vi "Word_Set_Page_Numbering.vi"(7 "Include total pages":bool, 8 "error in (no error)":errorcluster, 10 "alignment (right)":u16, 11 "report in":refnum<class "NI_report.lvclass">) -> (0 "error out":errorcluster, 3 "report out":refnum<class "NI_report.lvclass">)   [LabVIEW 2017, in "NI_ReportGenerationToolkit.lvlib"]
uses:
  <vilib>/addons/_office/NI_ReportGenerationToolkit.lvlib
  <vilib>/Utility/NIReport.llb/NI_report.lvclass
  <vilib>/Utility/NIReport.llb/Word/NI_Word.lvclass
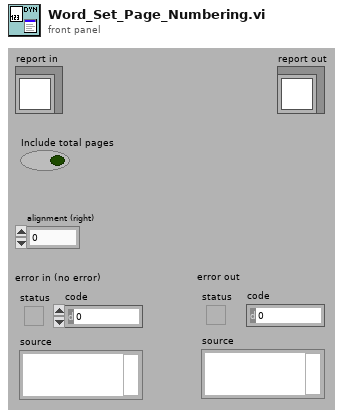
[diagram p1: front panel]
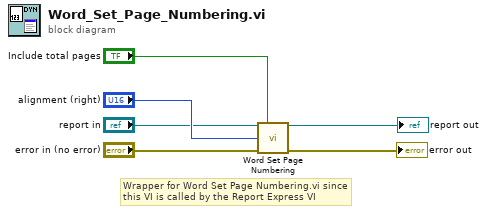
[diagram p0: block diagram]
diagram:
  # "Wrapper for Word Set Page Numbering.vi since\nthis VI is called by the Report Express VI"
  n1 = call <vilib>:"Word Set Page Numbering.vi"("report in"="report in", "include page x of n"="Include total pages", "alignment (right)"="alignment (right)", "error in (no error)"="error in (no error)") -> ("report out"=→"report out":refnum<class "NI_report.lvclass">, "error out"=→"error out":errorcluster)  [unwired: 10 in]
